vi "Actor Core.vi"(8 "error in":errorcluster, 11 "Image Acquisition in":refnum<class "Image Acquisition.lvclass">) -> (0 "error out":errorcluster, 3 "Actor out":refnum<class "Actor.lvclass">)   [LabVIEW 2019, in "Image Acquisition.lvlib" / "Image Acquisition.lvclass"]
doc: "(<B>Filename</B>: Actor Framework.lvlib:Actor.lvclass:Actor Core.vi)\n\nReceives messages to the actor, reacts to them, and initiates any error handling that may shut the actor down.\n\nDescendant classes may override this VI to append parallel tasks for the actor to complete while it handles messages. Overrides use the Call Parent Method node."
uses:
  Image Acquisition.lvclass
  <vilib>/ActorFramework/Actor/Actor.lvclass
  <vilib>/ActorFramework/Message Enqueuer/Message Enqueuer.lvclass
  Camera Controller/Camera Controller Messages/Child Handshake CC Msg/Child Handshake CC Msg.lvclass
  <vilib>/userdefined/High Color/IMAQdx.ctl
  <vilib>/vision/driver/IMAQdx.llb/IMAQdx Acquisition Mode.ctl
  <vilib>/vision/driver/IMAQdx.llb/IMAQdx Buffer Number Mode.ctl
  TypeDefs/Image Acquisition Parameters.ctl
  <vilib>/vision/Image Controls.llb/IMAQ Image.ctl
  TypeDefs/Initialize Data IA.ctl
  <resource>/objmgr/imaqdx.rc
  Camera Controller/Camera Controller Messages/Camera Information CC Msg/Camera Information CC Msg.lvclass
  <vilib>/event_ctls.llb/usereventprio.ctl
  Camera Controller/Camera Controller Messages/Get Image CC Msg/Get Image CC Msg.lvclass
  Camera Controller/Camera Controller Messages/State Acknowledgment CC Msg/State Acknowledgment CC Msg.lvclass
  C:/Program Files/National Instruments/LabVIEW 2019/vi.lib/ActorFramework/Actor/Actor.lvclass
panel:
  out "Image Acquisition ID":i32
  out "Acquired Image":T1(plugin-control)
  out "Camera Name":string
  out "Acquired Image Count":u64
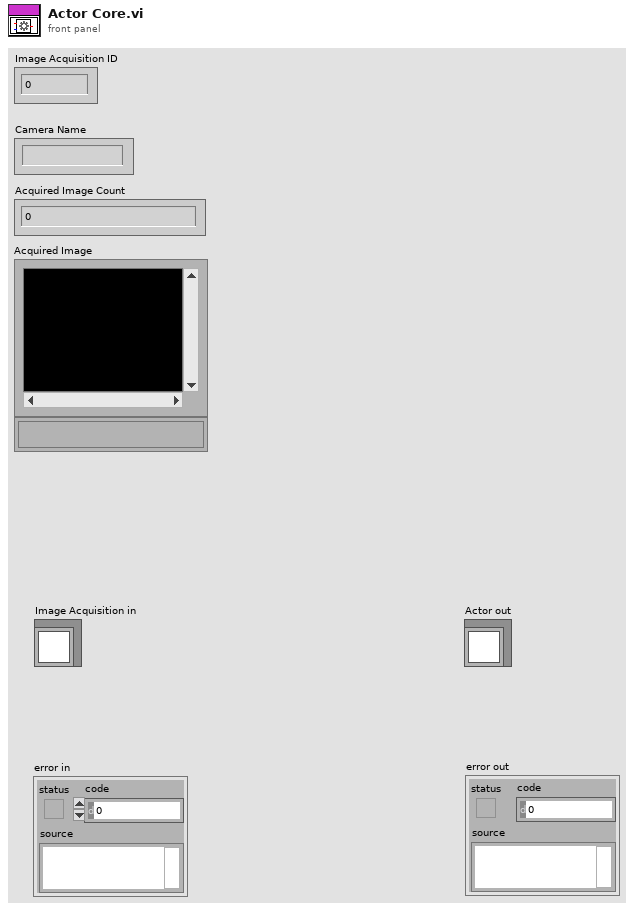
[diagram p1: front panel]
types:
  T1 = typedef "IMAQ Image.ctl" = refnum<image>
  T2 = typedef "Image Acquisition.lvlib/Image Acquisition.lvclass/Initialize Data IA.ctl" = cluster{"Core":cluster{"Current VI Reference":refnum<vi>, "Close Panel on Exit?":bool}, "IA JSON File Path":path, "Buffer Number":u64, "Missed Frame Count":i32, "Timeout":i32, "Image_Counter_CA":u64, "Imaqdx Session In":T3, "filenames":string[], "File path to read images":path, "Sequence":string, "IMAQ ring Buffer":T1[], "Buffer count":i32, "AOI":i32[], "Offline Images Ring Buffer":T1[], "ReceiverSequence":cluster{"ReceiverID":i32, "Index":i32}[], "Number Of Buffers":i32, "IMAQ Offline Image Buffer":T1[], "IMAQ Run image Buffer ":T1[], "Camera parameters":T4, "CurrentPartParameters":cluster{"Name":string, "ReceiverSequence":cluster{"ReceiverID":dbl, "Index":dbl}[], "AOI":i32[], "filePath":string}, "Exposure Time":u32, "File path @ Run":path, "State Ack":cluster{"State":string, "Status":string}}
  T3 = typedef "IMAQdx.ctl" = refnum<k21>
  T4 = typedef "Image Acquisition.lvlib/Image Acquisition.lvclass/Image Acquisition Parameters.ctl" = cluster{"Camera parameters":cluster{"Id":i32, "Type":string, "Model":string, "InterfaceType":string, "SerialNumber":string, "Timeout":i32, "NumberOfBuffers":i32, "AcquisitionTimeout":i32, "ImageName":string, "ColorCameraParam":cluster{"PixelFormat":string, "GammaEnable":bool, "GammaSelector":string, "BalanceRationSelector":string[], "BalanceRationRaw":i32[], "BalanceWhiteAuto":string, "LightSourceSelector":string}, "sessionID":T3, "Continuous?":T5, "Image Type":T6, "Buffer Number Mode (Next)":T7, "PartsList":cluster{"Name":string, "ReceiverSequence":cluster{"ReceiverID":dbl, "Index":dbl}[], "AOI":i32[], "filePath":string}[], "AOI ":i32[], "Default file path":path, "Offline":bool, "GeneralCameraConfig":cluster{"ActiveAttribute":string, "Value":string}[], "DefaultReceiverSequence":cluster{"ReceiverID":dbl, "Index":dbl}[], "Front Panel Open?":bool}, "PartName":string[]}
  T5 = typedef "NI_Vision_Acquisition_Software.lvlib/IMAQdx Acquisition Mode.ctl" = enum32{"One Shot", "Continuous"}
  T6 = typedef "Image Type" = u32
  T7 = typedef "NI_Vision_Acquisition_Software.lvlib/IMAQdx Buffer Number Mode.ctl" = enum32{"Next", "Last", "Buffer Number", "Every", "Last New"}
  T8 = typedef "Image Acquisition.lvlib/Image Acquisition.lvclass/Acquired Image Info.ctl" = cluster{"type":string, "Image Out":T1, "Buffer Number":u64, "Count":u64, "Buffer Count":u64}
  T9 = cluster{"Image out":T1, "Camera Location":string, "Count":u64, "RecieverSequence":cluster{"RecieverID":dbl, "Index":dbl}[]}
  T10 = enum32{"invalid app kind", "Development System", "Run Time System", "Student Edition", "Embedded LabVIEW", "Evaluation", "Custom"}
  T11 = enum32{"Invalid", "Standard", "Closed", "Hidden", "Minimized", "Maximized"}
  T12 = cluster{"Nested enqueuer":refnum<class "Message Enqueuer.lvclass">, "Clone name":string}
  T13 = cluster{"Camera Id":i32, "Camera Name":string, "Exposure Time":i32, "AOI":i32[]}
  T14 = typedef "usereventprio.ctl" = enum32{"high priority", "normal priority"}
  T15 = cluster{"ActiveAttribute":string, "Value":string}[]
  T16 = cluster{"ActiveAttribute":string, "Value":string}
  T17 = cluster{"Name":string, "ReceiverSequence":cluster{"ReceiverID":dbl, "Index":dbl}[], "AOI":i32[], "filePath":string}[]
  T18 = cluster{"Name":string, "ReceiverSequence":cluster{"ReceiverID":dbl, "Index":dbl}[], "AOI":i32[], "filePath":string}
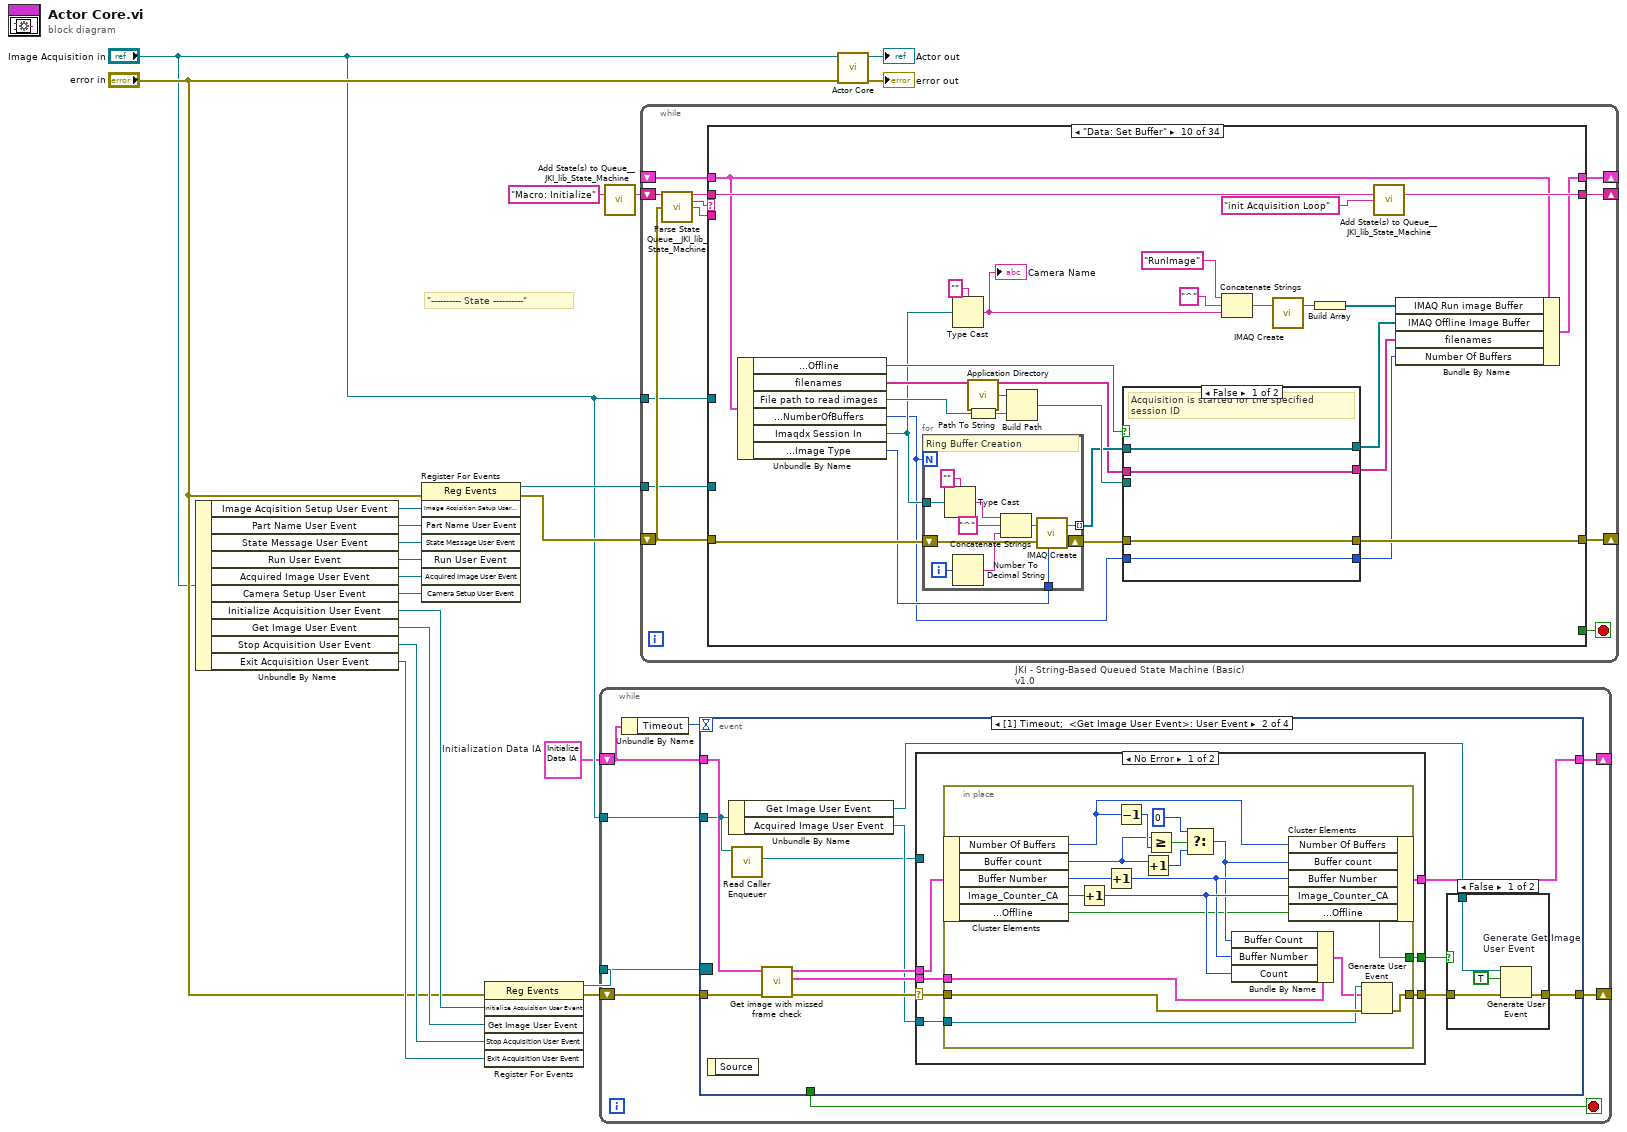
[diagram p0: block diagram]
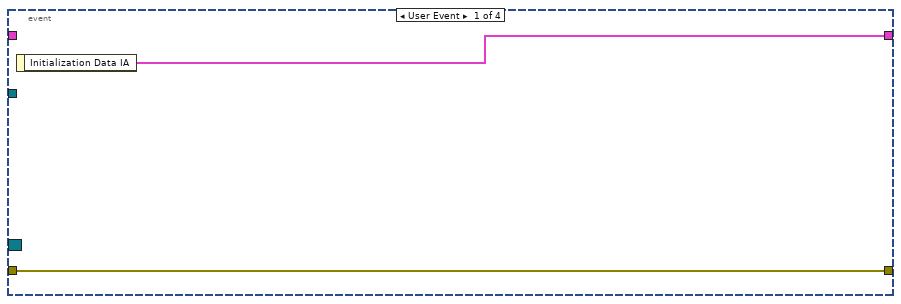
[diagram p2: hidden frame]
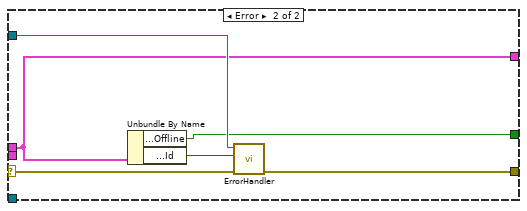
[diagram p4: hidden frame]
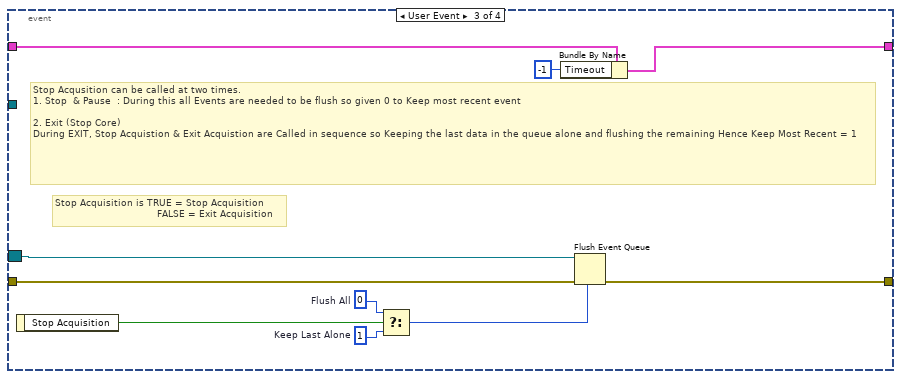
[diagram p5: hidden frame]
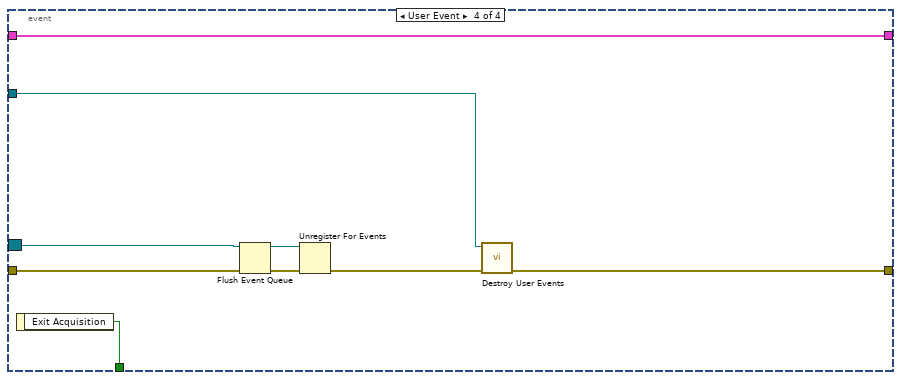
[diagram p6: hidden frame]
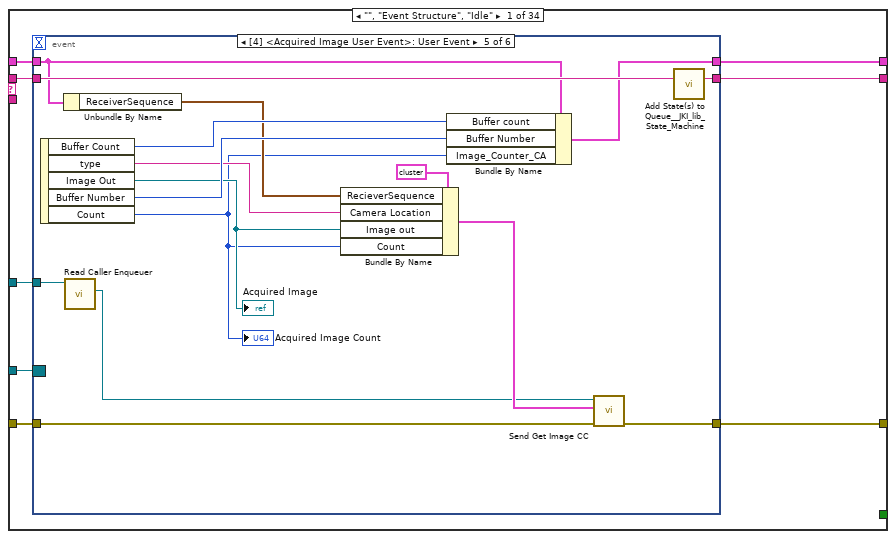
[diagram p7: hidden frame]
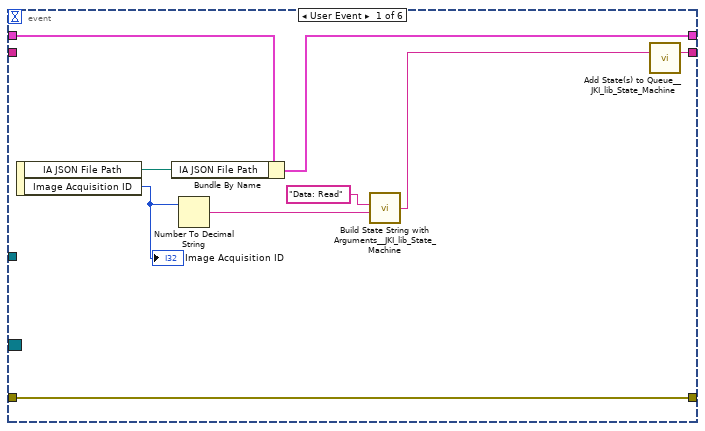
[diagram p8: hidden frame]
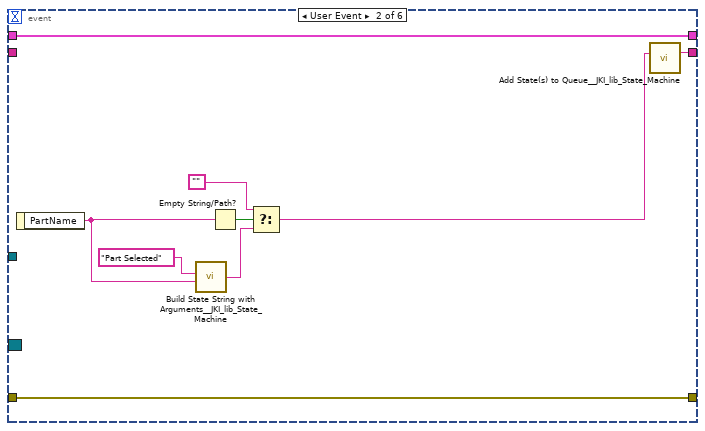
[diagram p9: hidden frame]
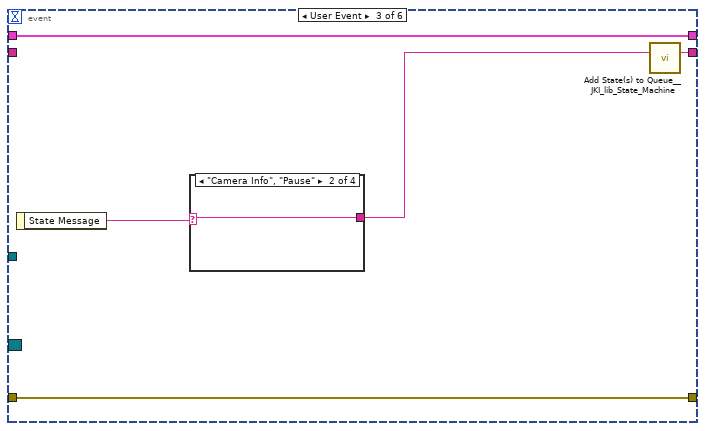
[diagram p10: hidden frame]
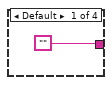
[diagram p11: hidden frame]
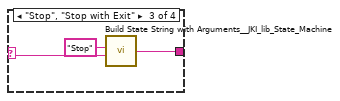
[diagram p12: hidden frame]
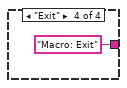
[diagram p13: hidden frame]
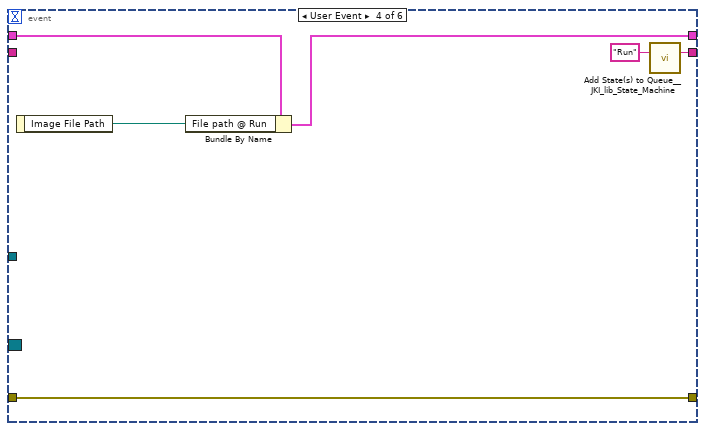
[diagram p14: hidden frame]
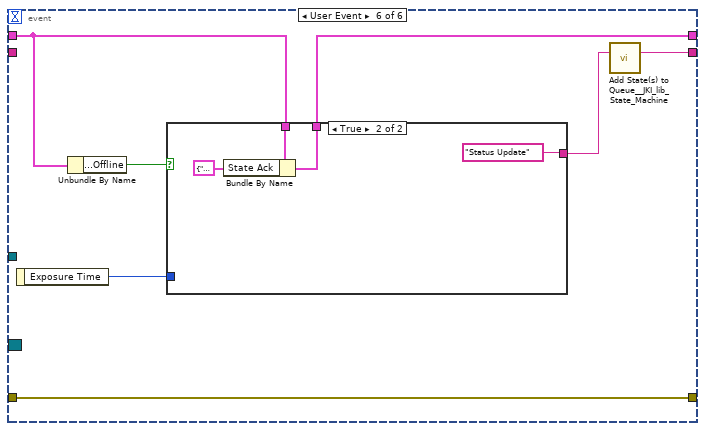
[diagram p15: hidden frame]
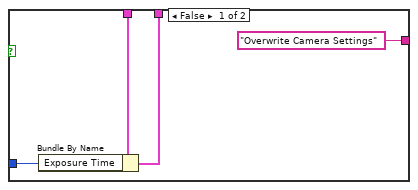
[diagram p16: hidden frame]
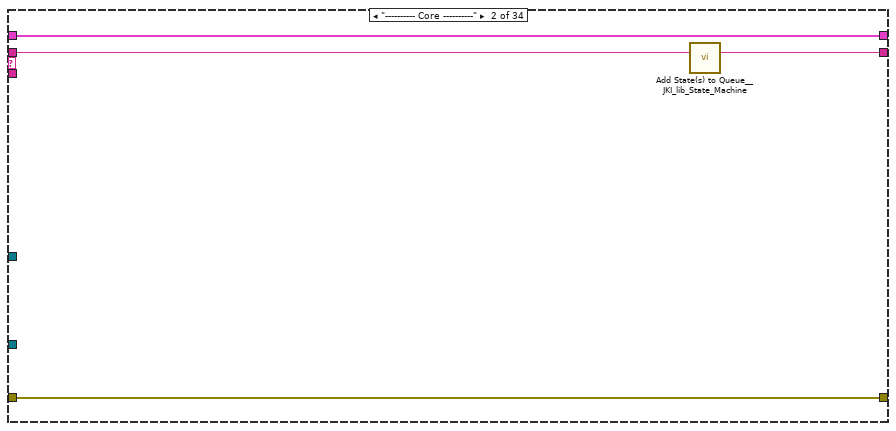
[diagram p17: hidden frame]
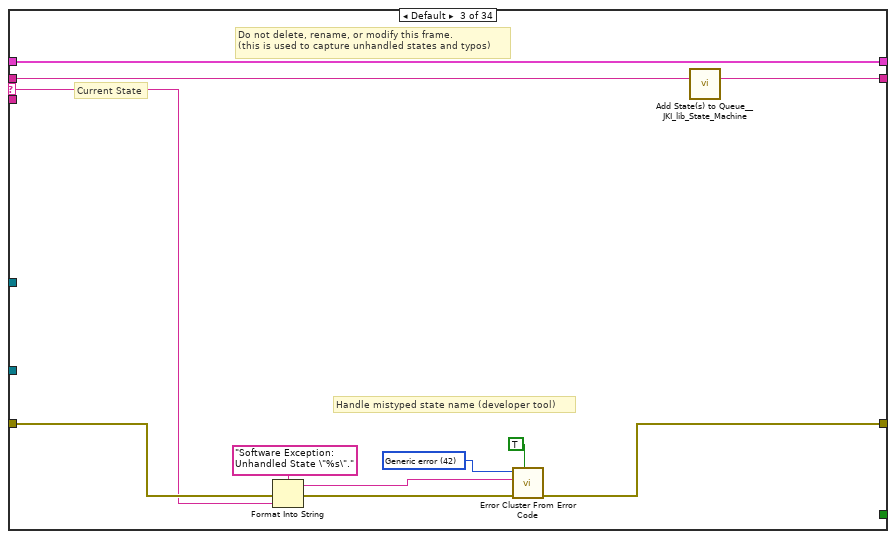
[diagram p18: hidden frame]
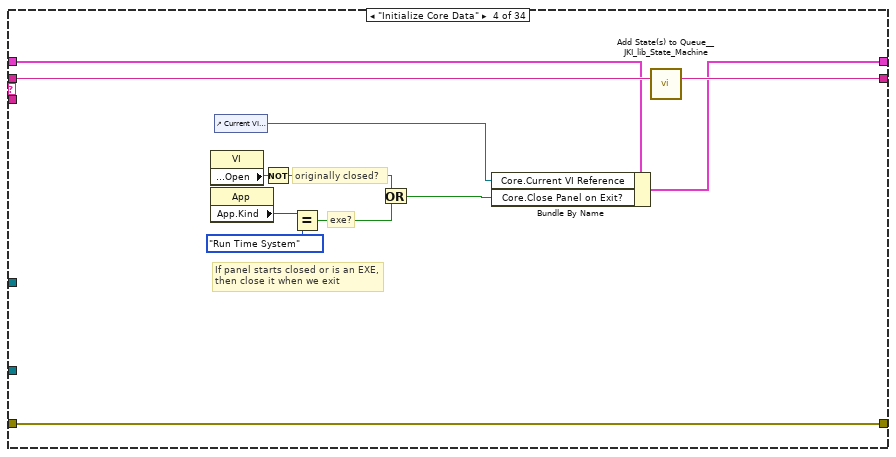
[diagram p19: hidden frame]
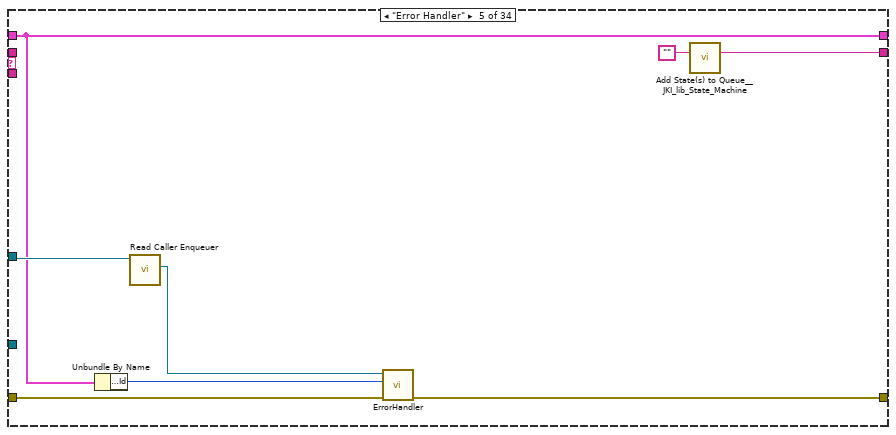
[diagram p20: hidden frame]
diagram:
  w1 = T2 {"Core"={"Current VI Reference"=refnum, "Close Panel on Exit?"=FALSE}, "IA JSON File Path"=path "", "Buffer Number"=0, "Missed Frame Count"=0, "Timeout"=-1, "Image_Counter_CA"=0, "Imaqdx Session In"="", "filenames"=[], "File path to read images"=path "", "Sequence"="", "IMAQ ring Buffer"=[], "Buffer count"=0, "AOI"=[], "Offline Images Ring Buffer"=[], "ReceiverSequence"=[], "Number Of Buffers"=0, "IMAQ Offline Image Buffer"=[], "IMAQ Run image Buffer "=[], "Camera parameters"={"Camera parameters"={"Id"=0, "Type"="", "Model"="", "InterfaceType"="", "SerialNumber"="", "Timeout"=0, "NumberOfBuffers"=0, "AcquisitionTimeout"=0, "ImageName"="", "ColorCameraParam"={"PixelFormat"="", "GammaEnable"=FALSE, "GammaSelector"="", "BalanceRationSelector"=[], "BalanceRationRaw"=[], "BalanceWhiteAuto"="", "LightSourceSelector"=""}, "sessionID"="", "Continuous?"=enum."One Shot", "Image Type"=0, "Buffer Number Mode (Next)"=enum."Next", "PartsList"=[{"Name"="", "ReceiverSequence"=[], "AOI"=[], "filePath"=""}], "AOI "=[], "Default file path"=path "", "Offline"=FALSE, "GeneralCameraConfig"=[], "DefaultReceiverSequence"=[], "Front Panel Open?"=FALSE}, "PartName"=[]}, "CurrentPartParameters"={"Name"="", "ReceiverSequence"=[], "AOI"=[], "filePath"=""}, "Exposure Time"=0, "File path @ Run"=path "", "State Ack"={"State"="", "Status"=""}}  # Initialization Data IA
  # "\"---------- State ----------\""
  n1 = Unbundle By Name("Image Acquisition in") -> ("Image Acqisition Setup User Event"=w17:refnum<user-event>, "Part Name User Event"=w16:refnum<user-event>, "State Message User Event"=w15:refnum<user-event>, "Run User Event"=w14:refnum<user-event>, "Acquired Image User Event"=w13:refnum<user-event>, "Camera Setup User Event"=w12:refnum<user-event>, "Initialize Acquisition User Event"=w9:refnum<user-event>, "Get Image User Event"=w8:refnum<user-event>, "Stop Acquisition User Event"=w7:refnum<user-event>, "Exit Acquisition User Event"=w6:refnum<user-event>)
  n2 = register-events(error in="error in", w17, w16, w15, w14, w13, w12) -> (reference out=w11:refnum<event-registration>, error out=w10:errorcluster)  [unwired: 1 in]
  n3 = register-events(error in="error in", w9, w8, w7, w6) -> (reference out=w5:refnum<event-registration>, error out=w3:errorcluster)  [unwired: 1 in]
  n4 = while {
    tunnel: w5 -> [w29]
    shift-right: [w26] -> _
    shift-left: w3 -> [w28]
    shift-right: [w27] -> _
    shift-left: w1 -> [w23]
    tunnel: "Image Acquisition in" -> [w24]
    stop <- w25 stop-if-true
    n5 = Unbundle By Name(w23) -> ("Timeout"=w22:i32)
    n6 = event shown="[1] Timeout;  <Get Image User Event>: User Event" {
      selector: w29 -> [_ _ w83 w93]
      dyn-events: _ -> [_ _ _ _]
      timeout: w22 -> [_ _ _ _]
      tunnel: w28 -> [w30 w44 w85 w94]
      tunnel: [w31 w32 w80 w98] -> w27
      tunnel: w23 -> [_ w43 w81 w98]
      tunnel: [w30 w37 w84 w91] -> w26
      tunnel: [_ _ _ w97] -> w25
      tunnel: w24 -> [_ w35 _ w90]
      event User Event {
        n7 = event-data() -> ("Initialization Data IA"=w31:T2)  [unwired: 1 in]
      }
      event Timeout; User Event {
        n8 = event-data() -> ()  [unwired: 1 in, 1 out]
        n9 = Unbundle By Name(w35) -> ("Get Image User Event"=w36:refnum<user-event>, "Acquired Image User Event"=w39:refnum<user-event>)
        n10 = call <vilib>:"Read Caller Enqueuer.vi"("Actor"=w35) -> ("Caller Enqueuer"=w34:refnum<class "Message Enqueuer.lvclass">)  [unwired: 10 in]
        n11 = call "Get image with missed frame check.vi"("error in"=w44, "Control IN"=w43) -> ("error out"=w42:errorcluster, "Get image Cluster"=w40:T8, "Controls Out"=w41:T2)  [unwired: 7 in]
        n12 = case shown="No Error" w42 {
          selector: w42 -> [w53 w79]
          tunnel: w41 -> [w56 w76]
          tunnel: w40 -> [w54 _]
          tunnel: [w55 w76] -> w32
          tunnel: w39 -> [w52 _]
          tunnel: [w51 w78] -> w38
          tunnel: w34 -> [_ w77]
          tunnel: [w50 w74] -> w33
          frame No Error {
            n13 = in-place {
              in-place-border: w54 -> [w58]
              in-place-border: w53 -> [w65]
              in-place-border: w52 -> [w63]
              in-place-border: [w64] -> w51
              in-place-border: [w57] -> w50
              n14 = in-place-cluster #1(w56) -> ("Number Of Buffers"=w66:i32, "Buffer count"=w69:i32, "Buffer Number"=w68:u64, "Image_Counter_CA"=w67:u64, "Camera parameters.Camera parameters.Offline"=w57:bool)
              n15 = Increment(x=w67) -> (x+1=w61:u64)
              n16 = Increment(x=w68) -> (x+1=w60:u64)
              n17 = Decrement(x=w66) -> (x-1=w72:i32)
              n18 = Increment(x=w69) -> (x+1=w70:i32)
              n19 = Greater Or Equal?(x=w69, y=w72) -> (x >= y?=w73:bool)
              n20 = Select(t=0, s=w73, f=w70) -> (s? t:f=w59:i32)
              n21 = Bundle By Name(cluster=w58, "Buffer Count"=w59, "Buffer Number"=w60, "Count"=w61) -> (w62:T8)
              n22 = in-place-cluster #1("Number Of Buffers"=w66, "Buffer count"=w59, "Buffer Number"=w60, "Image_Counter_CA"=w61, "Camera parameters.Camera parameters.Offline"=w57) -> (w55:T2)
              n23 = Generate User Event(user event=w63, event data cluster=w62, error in=w65) -> (error out=w64:errorcluster)  [unwired: 1 in, 1 out]
            }
          }
          frame Error {
            n24 = Unbundle By Name(w76) -> ("Camera parameters.Camera parameters.Offline"=w74:bool, "Camera parameters.Camera parameters.Id"=w75:i32)
            n25 = call "ErrorHandler.vi"("error in"=w79, "CameraID"=w75, "Caller Enqueuer"=w77) -> ("error out"=w78:errorcluster)  [unwired: 7 in, 1 out]
          }
        }
        n26 = case shown="False" w33 {
          tunnel: w38 -> [w48 w49]
          tunnel: [w47 w49] -> w37
          tunnel: w36 -> [w46 _]
          frame False {
            n27 = Generate User Event "Generate Get Image User Event"(user event=w46, event data cluster=TRUE ("event data"), error in=w48) -> (error out=w47:errorcluster)  [unwired: 1 in, 1 out]
          }
          frame True {
          }
        }
      }
      event User Event {
        w89 = 0  # Flush All
        w88 = 1  # Keep Last Alone
        # "Stop Acquisition is TRUE = Stop Acquisition\n                                  FALSE = Exit Acquisition"
        # "Stop Acqusition can be called at two times. \n1. Stop  & Pause  : During this all Events are needed to be flush so given 0 to Keep most recent event\n\n2. Exit (Stop Core)\nDuring EXIT, Stop Acquistion & Exit Acquistion are Called in sequence so Keeping the last data in the queue alone and flushing the remaining Hence Keep Most Recent = 1"
        n28 = event-data() -> ("Stop Acquisition"=w86:bool)  [unwired: 1 in]
        n29 = Select(t=w89, s=w86, f=w88) -> (s? t:f=w87:i32)
        n30 = Bundle By Name(cluster=w81, "Timeout"=-1) -> (w80:T2)
        n31 = Flush Event Queue(0:w83, 3:w85, 5:w87) -> (11:w84:errorcluster)  [unwired: 3 in, 2 out]
      }
      event User Event {
        n32 = event-data() -> ("Exit Acquisition"=w97:bool)  [unwired: 1 in]
        n33 = Flush Event Queue(0:w93, 3:w94) -> (8:w95:refnum<event-registration>, 11:w96:errorcluster)  [unwired: 4 in, 1 out]
        n34 = Unregister For Events(event registration refnum=w95, error in=w96) -> (error out=w92:errorcluster)
        n35 = call "Destroy User Events.vi"("error in (no error)"=w92, "Image Acquisition in"=w90) -> ("error out"=w91:errorcluster)  [unwired: 8 in, 1 out]
      }
    }
  }
  n36 = call <vilib>:"Add State(s) to Queue__JKI_lib_State_Machine.vi"("State(s) in (\"\")"="Macro: Initialize") -> ("States Out"=w19:string)  [unwired: 14 in]
  n37 = while "JKI - String-Based Queued State Machine (Basic) v1.0" {
    shift-right: [w103] -> _
    shift-left: _ -> [w102]
    shift-right: [w106] -> _
    shift-left: w10 -> [w101]
    shift-right: [w105] -> _
    shift-left: w19 -> [w107]
    tunnel: w11 -> [w100]
    tunnel: "Image Acquisition in" -> [w99]
    stop <- w104 stop-if-true
    n38 = call <vilib>:"Parse State Queue__JKI_lib_State_Machine.vi"("State Queue"=w107, "Error In (no error)"=w101) -> ("Remaining States"=w109:string, "Current State"=w110:string, "Arguments"=w108:string)  [unwired: 11 in]
    n39 = case shown="\"Data: Set Buffer\"" w110 {
      selector: w110 -> [_ _ w189 _ _ _ _ _ _ _ _ _ _ _ _ _ _ _ _ _ _ _ _ _ _ _ _ _ _ _ _ _ _ _]
      tunnel: w109 -> [w118 w188 w193 w211 _ w224 w228 w232 _ w288 w334 w350 w354 w360 w371 w397 w402 w414 w418 w430 w434 w449 _ _ _ w583 w627 w646 w680 w692 w700 w709 w717 w726]
      tunnel: w108 -> [_ _ _ _ _ _ _ _ w237 _ _ _ _ w355 w365 _ _ _ _ _ _ _ w459 _ _ w560 _ _ _ _ _ _ _ _]
      tunnel: w102 -> [w116 w185 w191 w202 w215 w222 w225 _ w235 w275 w330 w347 w352 w358 w367 w394 w399 w412 w415 w428 w431 w442 w454 w495 w544 w567 w624 w630 w663 w689 w694 w702 w715 w724]
      tunnel: [w115 w186 w195 w208 w213 w221 w226 w230 w239 w284 w324 w348 w351 w356 w368 w395 w400 w404 w416 w422 w432 w446 w456 w505 w545 w581 w625 w634 errorcluster {"status"=FALSE, "code"=0, "source"=""} ("error in (no error)") w690 w697 w705 w713 w722] -> w106
      tunnel: w101 -> [w114 w186 w194 w208 w218 w221 w226 w230 w240 w285 w331 w348 w351 w357 w369 w395 w400 w405 w416 w424 w432 w447 w457 w506 w546 w563 w625 w644 w672 w690 _ w706 w714 w723]
      tunnel: [w117 w187 w192 w210 w219 w223 w227 w231 w233 w287 w333 w349 w353 w359 w370 w396 w401 w413 w417 w429 w433 w448 w460 w507 w554 w582 w626 w645 w679 w691 w699 w708 w716 w725] -> w105
      tunnel: [_ _ _ _ _ TRUE _ _ _ _ _ _ _ _ _ _ _ _ _ _ _ _ _ _ _ _ _ _ _ _ _ _ _ _] -> w104
      tunnel: [w113 w185 w191 w209 w215 w222 w225 w229 w234 w274 w330 w347 w352 w358 w367 w394 w399 w412 w415 w428 w431 w442 w458 w494 w544 w580 w624 w629 w664 w689 w694 w702 w715 w724] -> w103
      tunnel: w100 -> [w112 _ _ _ _ _ _ _ _ _ _ _ _ _ _ _ _ w403 _ _ _ _ _ _ _ _ _ _ _ _ _ _ _ _]
      tunnel: w99 -> [w111 _ _ _ w217 _ _ _ _ _ _ _ _ _ _ _ _ _ _ w421 _ w445 _ _ w547 w564 _ w640 _ _ w696 w707 w712 w721]
      frame "", "Event Structure", "Idle" {
        n40 = event shown="[4] <Acquired Image User Event>: User Event" {
          selector: w112 -> [_ _ _ _ _ _]
          dyn-events: _ -> [_ _ _ _ _ _]
          timeout: _ -> [_ _ _ _ _ _]
          tunnel: w118 -> [_ _ _ _ w169 _]
          tunnel: [w127 w136 w141 w153 w168 w176] -> w117
          tunnel: w116 -> [w124 w134 w139 w150 w162 w171]
          tunnel: [w126 w135 w140 w152 w157 w175] -> w115
          tunnel: w114 -> [w126 w135 w140 w152 w158 w175]
          tunnel: [w123 w134 w139 w149 w161 w173] -> w113
          tunnel: w111 -> [_ _ _ _ w156 _]
          event User Event {
            n41 = event-data() -> ("IA JSON File Path"=w125:path, "Image Acquisition ID"=w122:i32)  [unwired: 1 in]
            "Image Acquisition ID" <- w122
            n42 = Bundle By Name(cluster=w124, "IA JSON File Path"=w125) -> (w123:T2)
            n43 = Number To Decimal String(number=w122) -> (decimal integer string=w121:string)  [unwired: 1 in]
            n44 = call <vilib>:"Build State String with Arguments__JKI_lib_State_Machine.vi"("Arguments (\"\")"=w121, "State"="Data: Read") -> ("State with Arguments"=w119:string)  [unwired: 4 in]
            n45 = call <vilib>:"Add State(s) to Queue__JKI_lib_State_Machine.vi"("State(s) in (\"\")"=w119) -> ("States Out"=w127:string)  [unwired: 14 in]
          }
          event User Event {
            n46 = event-data() -> ("PartName"=w133:string)  [unwired: 1 in]
            n47 = call <vilib>:"Build State String with Arguments__JKI_lib_State_Machine.vi"("Arguments (\"\")"=w133, "State"="Part Selected") -> ("State with Arguments"=w130:string)  [unwired: 4 in]
            n48 = Empty String/Path?(string/path=w133) -> (empty?=w132:bool)
            n49 = Select(t="", s=w132, f=w130) -> (s? t:f=w128:string)
            n50 = call <vilib>:"Add State(s) to Queue__JKI_lib_State_Machine.vi"("State(s) in (\"\")"=w128) -> ("States Out"=w136:string)  [unwired: 14 in]
          }
          event User Event {
            n51 = event-data() -> ("State Message"=w138:string)  [unwired: 1 in]
            n52 = case shown="\"Camera Info\", \"Pause\"" w138 {
              selector: w138 -> [_ w143 w146 _]
              tunnel: ["" w143 w144 "Macro: Exit" ("State with Arguments")] -> w137
              frame Default {
              }
              frame "Camera Info", "Pause" {
              }
              frame "Stop", "Stop with Exit" {
                n53 = call <vilib>:"Build State String with Arguments__JKI_lib_State_Machine.vi"("Arguments (\"\")"=w146, "State"="Stop") -> ("State with Arguments"=w144:string)  [unwired: 4 in]
              }
              frame "Exit" {
              }
            }
            n54 = call <vilib>:"Add State(s) to Queue__JKI_lib_State_Machine.vi"("State(s) in (\"\")"=w137) -> ("States Out"=w141:string)  [unwired: 14 in]
          }
          event User Event {
            n55 = event-data() -> ("Image File Path"=w151:path)  [unwired: 1 in]
            n56 = Bundle By Name(cluster=w150, "File path @ Run"=w151) -> (w149:T2)
            n57 = call <vilib>:"Add State(s) to Queue__JKI_lib_State_Machine.vi"("State(s) in (\"\")"="Run" ("State(s) in (\"\")")) -> ("States Out"=w153:string)  [unwired: 14 in]
          }
          event User Event {
            n58 = event-data() -> ("Buffer Count"=w164:u64, "type"=w165:string, "Image Out"=w166:T1, "Buffer Number"=w167:u64, "Count"=w154:u64)  [unwired: 1 in]
            "Acquired Image Count" <- w154
            "Acquired Image" <- w166
            n59 = Unbundle By Name(w162) -> ("ReceiverSequence"=w163:cluster{"ReceiverID":i32, "Index":i32}[])
            n60 = call <vilib>:"Read Caller Enqueuer.vi"("Actor"=w156) -> ("Caller Enqueuer"=w155:refnum<class "Message Enqueuer.lvclass">)  [unwired: 10 in]
            n61 = Bundle By Name(cluster=T9 {"Image out"=refnum, "Camera Location"="", "Count"=0, "RecieverSequence"=[]} ("Acquired Image Info"), "RecieverSequence"=w163, "Camera Location"=w165, "Image out"=w166, "Count"=w154) -> (w159:T9)
            n62 = Bundle By Name(cluster=w162, "Buffer count"=w164, "Buffer Number"=w167, "Image_Counter_CA"=w154) -> (w161:T2)
            n63 = call "Send Get Image CC.vi"("error in (no error)"=w158, "Acquired Image Info"=w159, "Message Enqueuer"=w155) -> ("error out"=w157:errorcluster)  [unwired: 7 in, 1 out]
            n64 = call <vilib>:"Add State(s) to Queue__JKI_lib_State_Machine.vi"("State(s) in (\"\")"=w169) -> ("States Out"=w168:string)  [unwired: 14 in]
          }
          event User Event {
            n65 = event-data() -> ("Exposure Time"=w174:i32)  [unwired: 1 in]
            n66 = Unbundle By Name(w171) -> ("Camera parameters.Camera parameters.Offline"=w170:bool)
            n67 = case shown="True" w170 {
              tunnel: w174 -> [w180 _]
              tunnel: [w179 w182] -> w173
              tunnel: ["Overwrite Camera Settings" "Status Update"] -> w172
              tunnel: w171 -> [w177 w183]
              frame False {
                n68 = Bundle By Name(cluster=w177, "Exposure Time"=w180) -> (w179:T2)
              }
              frame True {
                n69 = Bundle By Name(cluster=w183, "State Ack"=cluster{"State":string, "Status":string} {"State"="Setup", "Status"="Fail"}) -> (w182:T2)
              }
            }
            n70 = call <vilib>:"Add State(s) to Queue__JKI_lib_State_Machine.vi"("State(s) in (\"\")"=w172) -> ("States Out"=w176:string)  [unwired: 14 in]
          }
        }
      }
      frame "---------- Core ----------" {
        n71 = call <vilib>:"Add State(s) to Queue__JKI_lib_State_Machine.vi"("State(s) in (\"\")"=w188) -> ("States Out"=w187:string)  [unwired: 14 in]
      }
      frame Default {
        w198 = 42 items=["No error", "Argument error", "Memory is full", "Out of zone", "End of file", "File already open", "Generic file I/O error", "File not found", "File permission error", "Disk is full", "Duplicate path", "Too many files open", "System feature not enabled", "Resource file not found", "Cannot add resource", "Resource not found", "Image not found", "Image memory error", "Pen does not exist", "Config type invalid", "Config token not found", "Config parse error", "Config memory error", "Bad external code format", "Bad external code offset", "External code not present", "Null window", "Destroy window error", "Null menu", "Print aborted", "Bad print record", "Print driver error", "Windows error during printing", "Memory error during printing", "Print dialog error", "Generic print error", "Invalid device refnum", "Device not found", "Device parameter error", "Device unit error", "Cannot open device", "Device call aborted", "Generic error", "Cancelled by user", "Object ID too low", "Object ID too high", "Object not in heap", "Unknown heap", "Unknown object (invalid DefProc)", "Unknown object (DefProc not in table)", "Message out of range", "Invalid (null) method", "Unknown message", "Manager call not supported", "Bad address", "Network operation in progress", "Network operation timed out", "Connection is busy", "Network attribute not supported", "Network error", "Address in use", "System out of memory", "Connection aborted", "Connection refused", "Not connected", "Already connected", "Connection closed", "Initialization error (interapplication manager)", "Bad occurrence", "Wait on unbound occurrence handler", "Occurrence queue overflow", "Datalog type conflict", "Unused", "Unrecognized type (interapplication manager)", "Memory corrupt", "Failed to make temporary DLL", "Old CIN version", "Drag socket not found", "Failed to load drop-object", "Failed to register OLE object", "Failed to release OLE object", "Format specifier type mismatch", "Unknown format specifier", "Too few format specifiers", "Too many format specifiers", "Scan failed", "Newer CIN version", "Error converting to variant", "Runtime menu error", "Password tampered", "Variant attribute not found", "Incompatible variant data type", "Event data is not available", "Event Store is not present", "Occurrence is not found", "Event Queue is not created", "Event info is not available", "Refnum passed is NULL", "Error retrieving Class GUID", "Error retrieving CoClass GUID", "Error retrieving TypeLib GUID.", "Bad built application magic bytes.", "Specific driver is different from the specific driver associated with the Logical Name.", "There is no session opened to the class driver.", "Max Error", "MAX - Error with config objects", "MAX - Error loading configuration", "MAX - Group not supported"]
        # "Current State"
        # "Do not delete, rename, or modify this frame.\n(this is used to capture unhandled states and typos)"
        # "Handle mistyped state name (developer tool)"
        n72 = Format Into String(format string="Software Exception: Unhandled State \"%s\"." ("message"), error in=w194, w189) -> (resulting string=w197:string, error out=w196:errorcluster)  [unwired: 1 in]
        n73 = call <vilib>:"Error Cluster From Error Code.vi"("show call chain? (False)"=TRUE, "error in (no error)"=w196, "error message (\"\")"=w197, "error code (0)"=w198) -> ("error out"=w195:errorcluster)  [unwired: 5 in]
        n74 = call <vilib>:"Add State(s) to Queue__JKI_lib_State_Machine.vi"("State(s) in (\"\")"=w193) -> ("States Out"=w192:string)  [unwired: 14 in]
      }
      frame "Initialize Core Data" {
        # "originally closed?"
        # "exe?"
        # "If panel starts closed or is an EXE, then close it when we exit"
        n75 = property class="VI"() -> ("Front Panel.Open"=w207:bool)  [unwired: 2 in, 2 out]
        n76 = property class="App"() -> ("App.Kind"=w206:T10)  [unwired: 2 in, 2 out]
        n77 = control-ref of="Current VI Reference"() -> (w200:refnum<vi>)
        n78 = Not(x=w207) -> (.not. x?=w204:bool)
        n79 = Equal?(x=w206, y=T10."Run Time System" ("Application:Kind")) -> (x = y?=w203:bool)
        n80 = Or(x=w204, y=w203) -> (x .or. y?=w201:bool)
        n81 = Bundle By Name(cluster=w202, "Core.Current VI Reference"=w200, "Core.Close Panel on Exit?"=w201) -> (w209:T2)
        n82 = call <vilib>:"Add State(s) to Queue__JKI_lib_State_Machine.vi"("State(s) in (\"\")"=w211) -> ("States Out"=w210:string)  [unwired: 14 in]
      }
      frame "Error Handler" {
        n83 = Unbundle By Name(w215) -> ("Camera parameters.Camera parameters.Id"=w214:i32)
        n84 = call <vilib>:"Read Caller Enqueuer.vi"("Actor"=w217) -> ("Caller Enqueuer"=w216:refnum<class "Message Enqueuer.lvclass">)  [unwired: 10 in]
        n85 = call "ErrorHandler.vi"("error in"=w218, "CameraID"=w214, "Caller Enqueuer"=w216) -> ("error out"=w213:errorcluster)  [unwired: 7 in, 1 out]
        n86 = call <vilib>:"Add State(s) to Queue__JKI_lib_State_Machine.vi"("State(s) in (\"\")"="") -> ("States Out"=w219:string)  [unwired: 14 in]
      }
      frame "Exit" {
        # "Do not put any code in this frame.\n(No errors that occur here will be handled.)"
        n87 = call <vilib>:"Add State(s) to Queue__JKI_lib_State_Machine.vi"("State(s) in (\"\")"=w224) -> ("States Out"=w223:string)  [unwired: 14 in]
      }
      frame "---------- Data ----------" {
        # "Do not put any code in this frame.\n(It is a separator no-op. You can make a copy of this frame to create a new Data frame)"
        n88 = call <vilib>:"Add State(s) to Queue__JKI_lib_State_Machine.vi"("State(s) in (\"\")"=w228) -> ("States Out"=w227:string)  [unwired: 14 in]
      }
      frame "Data: Initialize" {
        w229 = T2 {"Core"={"Current VI Reference"=refnum, "Close Panel on Exit?"=FALSE}, "IA JSON File Path"=path "", "Buffer Number"=0, "Missed Frame Count"=0, "Timeout"=-1, "Image_Counter_CA"=0, "Imaqdx Session In"="", "filenames"=[], "File path to read images"=path "", "Sequence"="", "IMAQ ring Buffer"=[], "Buffer count"=0, "AOI"=[], "Offline Images Ring Buffer"=[], "ReceiverSequence"=[], "Number Of Buffers"=0, "IMAQ Offline Image Buffer"=[], "IMAQ Run image Buffer "=[], "Camera parameters"={"Camera parameters"={"Id"=0, "Type"="", "Model"="", "InterfaceType"="", "SerialNumber"="", "Timeout"=0, "NumberOfBuffers"=0, "AcquisitionTimeout"=0, "ImageName"="", "ColorCameraParam"={"PixelFormat"="", "GammaEnable"=FALSE, "GammaSelector"="", "BalanceRationSelector"=[], "BalanceRationRaw"=[], "BalanceWhiteAuto"="", "LightSourceSelector"=""}, "sessionID"="", "Continuous?"=enum."One Shot", "Image Type"=0, "Buffer Number Mode (Next)"=enum."Next", "PartsList"=[{"Name"="", "ReceiverSequence"=[], "AOI"=[], "filePath"=""}], "AOI "=[], "Default file path"=path "", "Offline"=FALSE, "GeneralCameraConfig"=[], "DefaultReceiverSequence"=[], "Front Panel Open?"=FALSE}, "PartName"=[]}, "CurrentPartParameters"={"Name"="", "ReceiverSequence"=[], "AOI"=[], "filePath"=""}, "Exposure Time"=0, "File path @ Run"=path "", "State Ack"={"State"="", "Status"=""}}  # Initialization Data IA
        n89 = call <vilib>:"Add State(s) to Queue__JKI_lib_State_Machine.vi"("State(s) in (\"\")"=w232) -> ("States Out"=w231:string)  [unwired: 14 in]
      }
      frame "Data: Read" {
        n90 = Unbundle By Name(w235) -> ("IA JSON File Path"=w238:path)
        n91 = call "ReadJSONImageAcquisitionParameters.vi"("error in"=w240, "Camera ID"=w237, "file path (use dialog)"=w238) -> ("error out"=w239:errorcluster, "Camera parameters"=w236:T4)  [unwired: 7 in]
        n92 = in-place {
          in-place-border: w236 -> [w260]
          in-place-border: [w252] -> w233
          n93 = in-place-cluster #2(w235) -> ()  [unwired: 6 out]
          n94 = in-place-cluster #3(w236) -> ("Camera parameters.GeneralCameraConfig"=w242:T15, "Camera parameters.sessionID"=w246:T3, "Camera parameters.Front Panel Open?"=w251:bool, "Camera parameters.Offline"=w250:bool, "Camera parameters.Default file path"=w249:path, "Camera parameters.DefaultReceiverSequence"=w248:cluster{"ReceiverID":dbl, "Index":dbl}[], "Camera parameters.AOI"=w247:i32[])
          n95 = Index Array(array=w242, index=2) -> (element=w244:T16)
          n96 = Unbundle By Name(w244) -> ("Value"=w243:string)
          n97 = Select(t="UI: Front Panel State >> Open ", s=w251, f="UI: Front Panel State >> Close ") -> (s? t:f=w255:string)
          n98 = Decimal String To Number(string=w243) -> (number=w241:i32)  [unwired: 2 in, 1 out]
          n99 = Select(t="", s=w250, f="Set Camera Properties") -> (s? t:f=w254:string)
          n100 = in-place-cluster #3("Camera parameters.GeneralCameraConfig"=w242, "Camera parameters.sessionID"=w246, "Camera parameters.Front Panel Open?"=w251, "Camera parameters.Offline"=w250, "Camera parameters.Default file path"=w249, "Camera parameters.DefaultReceiverSequence"=w248, "Camera parameters.AOI"=w247) -> ()  [unwired: 1 out]
          n101 = in-place-cluster #2("File path to read images"=w249, "ReceiverSequence"=w248, "AOI"=w247, "Camera parameters"=w260, "Imaqdx Session In"=w246, "Exposure Time"=w241) -> (w234:T2)
          n102 = call <vilib>:"Add State(s) to Queue__JKI_lib_State_Machine.vi"("State(s) in Front (\"\")"=w255, "State(s) in (\"\")"=w254, "State(s) at Back (\"\")"="Data: Set Buffer" ("State(s) in (\"\")")) -> ("States Out"=w252:string)  [unwired: 12 in]
        }
      }
      frame "Data: Set Buffer" {
        n103 = Unbundle By Name(w275) -> ("Camera parameters.Camera parameters.Offline"=w278:bool, "filenames"=w277:string[], "File path to read images"=w281:path, "Camera parameters.Camera parameters.NumberOfBuffers"=w262:i32, "Imaqdx Session In"=w267:T3, "Camera parameters.Camera parameters.Image Type"=w276:T6)
        n104 = for {
          N: w262 -> [_]
          shift-right: [w320] -> w286
          shift-left: w285 -> [w321]
          tunnel: w267 -> [w317]
          tunnel: w276 -> [w312]
          tunnel: [w311] -> w279 mode=indexing
          i -> [w314]
          # "Ring Buffer Creation"
          n105 = Type Cast(type="" ("Camera Location"), x=w317) -> (*(type *) &x=w319:string)
          n106 = Number To Decimal String(number=w314) -> (decimal integer string=w313:string)  [unwired: 1 in]
          n107 = Concatenate Strings(w319, "^" ("string"), w313) -> (w315:string)
          n108 = call "IMAQ Create"("Image Name"=w315, "Image Type"=w312, "error in (no error)"=w321) -> ("New Image"=w311:T1, "error out"=w320:errorcluster)  [unwired: 2 in]
        }
        n109 = Type Cast(type="" ("Camera Location"), x=w267) -> (*(type *) &x=w265:string)
        "Camera Name" <- w265
        n110 = call <vilib>:"Application Directory.vi"() -> ("Application Directory"=w283:path)
        n111 = Path To String(path=w281) -> (string=w282:string)
        n112 = Build Path(base path=w283, name or relative path=w282) -> (appended path=w280:path)
        n113 = case shown="False" w278 {
          tunnel: w286 -> [w292 w302]
          tunnel: [w292 w297] -> w284
          tunnel: w280 -> [_ w300]
          tunnel: w277 -> [w290 _]
          tunnel: w279 -> [w291 w294]
          tunnel: [w291 w296] -> w269
          tunnel: [w290 w295] -> w271
          tunnel: [w289 w293] -> w261
          tunnel: w262 -> [w289 _]
          frame False {
            # "Acquisition is started for the specified session ID"
          }
          frame True {
            # "database is accessed for the image names and sorted"
            n114 = List Folder(path=w300, error in=w302) -> (filenames=w301:string[], error out=w298:errorcluster)  [unwired: 2 in, 2 out]
            n115 = Sort 1D Array ("Sort Array")(array=w301) -> (sorted array=w299:string[])
            n116 = for {
              tunnel: w300 -> [w310]
              tunnel: w299 -> [w306] mode=indexing
              shift-right: [w309] -> w297
              shift-left: w298 -> [w305]
              tunnel: [w307] -> w296 mode=indexing
              tunnel: [w306] -> w295 mode=indexing
              tunnel: w294 -> [w304] mode=indexing
              tunnel: [w303] -> w293
              i -> [w303]
              n117 = Build Path(base path=w310, name or relative path=w306) -> (appended path=w308:path)
              n118 = call "IMAQ ReadFile"("File Path"=w308, "error in (no error)"=w305, "Image"=w304) -> ("error out"=w309:errorcluster, "Image Out"=w307:T1)  [unwired: 4 in, 3 out]
            }
          }
        }
        n119 = Concatenate Strings("RunImage" ("Image Name"), "^" ("string"), w265) -> (w263:string)
        n120 = call "IMAQ Create"("Image Name"=w263) -> ("New Image"=w273:T1)  [unwired: 4 in, 1 out]
        n121 = Build Array(w273) -> (w272:T1[])
        n122 = call <vilib>:"Add State(s) to Queue__JKI_lib_State_Machine.vi"("State(s) in (\"\")"=w288, "State(s) at Back (\"\")"="init Acquisition Loop" ("State(s) at Back (\"\")")) -> ("States Out"=w287:string)  [unwired: 13 in]
        n123 = Bundle By Name(cluster=w275, "IMAQ Run image Buffer"=w272, "IMAQ Offline Image Buffer"=w269, "filenames"=w271, "Number Of Buffers"=w261) -> (w274:T2)
      }
      frame "Data: Cleanup" {
        n124 = Unbundle By Name(w330) -> ("IMAQ Offline Image Buffer"=w323:T1[], "IMAQ Run image Buffer"=w322:T1[], "Imaqdx Session In"=w328:T3, "Camera parameters.Camera parameters.Offline"=w327:bool, "Core.Current VI Reference"=w332:refnum<vi>)
        n125 = Close Reference(reference=w332, error in (no error)=w331) -> (error out=w329:errorcluster)
        n126 = case shown="False" w327 {
          tunnel: w329 -> [w341 w346]
          tunnel: w328 -> [w342 _]
          tunnel: [w344 w346] -> w325
          frame False {
            n127 = call <vilib>:"IMAQdx Unconfigure Acquisition.vi"("error in"=w341, "Session In"=w342) -> ("error out"=w345:errorcluster, "Session Out"=w343:T3)  [unwired: 8 in]
            n128 = call <vilib>:"IMAQdx Close Camera.vi"("error in"=w345, "Session In"=w343) -> ("error out"=w344:errorcluster)  [unwired: 9 in]
          }
          frame True {
          }
        }
        n129 = call <vilib>:"Add State(s) to Queue__JKI_lib_State_Machine.vi"("State(s) in (\"\")"=w334) -> ("States Out"=w333:string)  [unwired: 14 in]
        n130 = for {
          tunnel: [w340] -> w326
          tunnel: w322 -> [w339] mode=indexing
          tunnel: w325 -> [w338]
          n131 = call "IMAQ Dispose"("Image"=w339, "error in (no error)"=w338) -> ("error out"=w340:errorcluster)  [unwired: 4 in]
        }
        n132 = for {
          tunnel: w326 -> [w337]
          tunnel: w323 -> [w335] mode=indexing
          tunnel: [w336] -> w324
          tunnel: [w335] -> _ mode=indexing
          n133 = call "IMAQ Dispose"("Image"=w335, "error in (no error)"=w337) -> ("error out"=w336:errorcluster)  [unwired: 4 in]
        }
      }
      frame "---------- UI ----------" {
        n134 = call <vilib>:"Add State(s) to Queue__JKI_lib_State_Machine.vi"("State(s) in (\"\")"=w350) -> ("States Out"=w349:string)  [unwired: 14 in]
      }
      frame "UI: Initialize" {
        # "Initialize the User Interface, here.\n(this is called automatically, by the Macro: Init)"
        n135 = call <vilib>:"Add State(s) to Queue__JKI_lib_State_Machine.vi"("State(s) in (\"\")"=w354) -> ("States Out"=w353:string)  [unwired: 14 in]
      }
      frame "UI: Cursor Set" {
        # "Argument"
        # "Set and Unset Cursor Busy.\n(Usage: \"UI: Cursor Set >> Busy|Idle\")"
        n136 = case shown="\"Idle\", Default" w355 {
          tunnel: w357 -> [w362 w364]
          tunnel: [w361 w363] -> w356
          frame "Idle", Default {
            n137 = call <vilib>:"Unset Busy.vi"("error in (no error)"=w362) -> ("error out"=w361:errorcluster)  [unwired: 10 in]
          }
          frame "Busy" {
            n138 = call <vilib>:"Set Busy.vi"("error in (no error)"=w364) -> ("error out"=w363:errorcluster)  [unwired: 9 in, 1 out]
          }
        }
        n139 = call <vilib>:"Add State(s) to Queue__JKI_lib_State_Machine.vi"("State(s) in (\"\")"=w360) -> ("States Out"=w359:string)  [unwired: 14 in]
      }
      frame "UI: Front Panel State" {
        # "Argument"
        # "Set Front Panel Open or Closed\n(Usage: \"UI: Front Panel State >> Open|Close\")"
        n140 = Unbundle By Name(w367) -> ("Core.Current VI Reference"=w366:refnum<vi>)
        n141 = case shown="\"Open\", Default" w365 {
          tunnel: w369 -> [w375 w388]
          tunnel: [w377 w389] -> w368
          tunnel: w366 -> [w376 w386]
          frame "Open", Default {
            n142 = property class="VI"(reference=w376, error in=w375) -> (reference out=w373:refnum<vi>, error out=w374:errorcluster, "Front Panel.Open"=w372:bool)
            n143 = case shown="False" w372 {
              tunnel: [w380 w383] -> w377
              tunnel: w374 -> [w379 w383]
              tunnel: w373 -> [w378 _]
              frame False {
                n144 = invoke class="VI" method="FP.Open"(reference=w378, error in=w379, "Activate"=TRUE, "State"=T11."Standard") -> (error out=w380:errorcluster)  [unwired: 1 in, 4 out]
              }
              frame True {
              }
            }
          }
          frame "Close" {
            n145 = property class="VI"(reference=w386, error in=w388) -> (reference out=w385:refnum<vi>, error out=w387:errorcluster, "Front Panel.Open"=w384:bool)
            n146 = case shown="True" w384 {
              tunnel: [w390 w393] -> w389
              tunnel: w387 -> [w390 w392]
              tunnel: w385 -> [_ w391]
              frame False {
              }
              frame True {
                n147 = invoke class="VI" method="FP.Close"(reference=w391, error in=w392) -> (error out=w393:errorcluster)  [unwired: 1 in, 2 out]
              }
            }
          }
        }
        n148 = call <vilib>:"Add State(s) to Queue__JKI_lib_State_Machine.vi"("State(s) in (\"\")"=w371) -> ("States Out"=w370:string)  [unwired: 14 in]
      }
      frame "---------- Macro ----------" {
        # "Do not put any code in this frame.\n(It is a separator no-op. You can make a copy of this frame to create a new Macro frame)"
        n149 = call <vilib>:"Add State(s) to Queue__JKI_lib_State_Machine.vi"("State(s) in (\"\")"=w397) -> ("States Out"=w396:string)  [unwired: 14 in]
      }
      frame "Macro: Initialize" {
        n150 = call <vilib>:"Add State(s) to Queue__JKI_lib_State_Machine.vi"("State(s) in Front (\"\")"="Data: Initialize\nInitialize Core Data\ninit Acquisition Loop\nLaunch Handshake", "State(s) in (\"\")"=w402) -> ("States Out"=w401:string)  [unwired: 13 in]
      }
      frame "Macro: Exit" {
        n151 = Unbundle By Name(w412) -> ("Core.Close Panel on Exit?"=w411:bool)
        n152 = Flush Event Queue(0:w403, 3:w405) -> (11:w404:errorcluster)  [unwired: 4 in, 2 out]
        n153 = Select(t="UI: Front Panel State >> Close", s=w411, f="") -> (s? t:f=w406:string)
        n154 = call <vilib>:"Add State(s) to Queue__JKI_lib_State_Machine.vi"("State(s) in (\"\")"=w406, "State(s) at Back (\"\")"="Exit Acquisition Loop \nData: Cleanup\nExit") -> ("States Out"=w407:string)  [unwired: 13 in]
        n155 = call <vilib>:"Add State(s) to Queue__JKI_lib_State_Machine.vi"("State(s) in Front (\"\")"=w407, "State(s) in (\"\")"=w414) -> ("States Out"=w413:string)  [unwired: 13 in]
      }
      frame "---------- Launch ----------" {
        n156 = call <vilib>:"Add State(s) to Queue__JKI_lib_State_Machine.vi"("State(s) in (\"\")"=w418) -> ("States Out"=w417:string)  [unwired: 14 in]
      }
      frame "Launch Handshake" {
        n157 = call <vilib>:"Read Self Enqueuer.vi"("Actor"=w421) -> ("Self Enqueuer"=w426:refnum<class "Message Enqueuer.lvclass">)  [unwired: 10 in]
        n158 = call <vilib>:"Read Caller Enqueuer.vi"("Actor"=w421) -> ("Caller Enqueuer"=w420:refnum<class "Message Enqueuer.lvclass">)  [unwired: 10 in]
        n159 = property class="VI"(error in=w424) -> (error out=w423:errorcluster, "Name"=w427:string)  [unwired: 1 in, 1 out]
        n160 = Bundle By Name(cluster=T12 {"Nested enqueuer"=refnum, "Clone name"=""} ("Child launch Check"), "Nested enqueuer"=w426, "Clone name"=w427) -> (w419:T12)
        n161 = call "Send Child Handshake CC.vi"("error in (no error)"=w423, "Child Core Data"=w419, "Message Enqueuer"=w420) -> ("error out"=w422:errorcluster)  [unwired: 7 in, 1 out]
        n162 = call <vilib>:"Add State(s) to Queue__JKI_lib_State_Machine.vi"("State(s) in (\"\")"=w430) -> ("States Out"=w429:string)  [unwired: 14 in]
      }
      frame "---------- State ----------" {
        n163 = call <vilib>:"Add State(s) to Queue__JKI_lib_State_Machine.vi"("State(s) in (\"\")"=w434) -> ("States Out"=w433:string)  [unwired: 14 in]
      }
      frame "Camera Info" {
        n164 = call <vilib>:"Read Caller Enqueuer.vi"("Actor"=w445) -> ("Caller Enqueuer"=w444:refnum<class "Message Enqueuer.lvclass">)  [unwired: 10 in]
        n165 = Unbundle By Name(w442) -> ("ReceiverSequence"=w438:cluster{"ReceiverID":i32, "Index":i32}[], "Camera parameters.Camera parameters.Type"=w441:string, "Exposure Time"=w435:u32, "AOI"=w440:i32[])
        n166 = Index Array(array=w438) -> (element=w439:cluster{"ReceiverID":i32, "Index":i32})  [unwired: 1 in]
        n167 = Unbundle By Name(w439) -> ("Index"=w437:i32)
        n168 = Bundle By Name(cluster=T13 {"Camera Id"=0, "Camera Name"="", "Exposure Time"=0, "AOI"=[]} ("Camera Information"), "Camera Id"=w437, "Camera Name"=w441, "Exposure Time"=w435, "AOI"=w440) -> (w436:T13)
        n169 = call "Send Camera Information CC.vi"("error in (no error)"=w447, "Camera Information"=w436, "Message Enqueuer"=w444) -> ("error out"=w446:errorcluster)  [unwired: 7 in, 1 out]
        n170 = call <vilib>:"Add State(s) to Queue__JKI_lib_State_Machine.vi"("State(s) in (\"\")"=w449) -> ("States Out"=w448:string)  [unwired: 14 in]
      }
      frame "Part Selected" {
        n171 = in-place {
          in-place-border: w459 -> [w478]
          in-place-border: w457 -> [w468]
          in-place-border: [w465] -> w456
          w469 = 0
          n172 = in-place-cluster #4(w454) -> ("Camera parameters.Camera parameters.PartsList"=w476:T17, "Camera parameters.PartName"=w475:string[], "IMAQ Run image Buffer"=w464:T1[], "IMAQ Offline Image Buffer"=w463:T1[], "Imaqdx Session In"=w462:T3, "Camera parameters.Camera parameters.Offline"=w461:bool)  [unwired: 7 out]
          n173 = Search 1D Array(1D array=w475, element=w478) -> (index of element=w477:i32)  [unwired: 1 in]
          n174 = case shown="False" w461 {
            tunnel: w468 -> [w485 w490]
            tunnel: w462 -> [w486 _]
            tunnel: [w488 w490] -> w467
            frame False {
              n175 = call <vilib>:"IMAQdx Unconfigure Acquisition.vi"("error in"=w485, "Session In"=w486) -> ("error out"=w489:errorcluster, "Session Out"=w487:T3)  [unwired: 8 in]
              n176 = call <vilib>:"IMAQdx Close Camera.vi"("error in"=w489, "Session In"=w487) -> ("error out"=w488:errorcluster)  [unwired: 9 in]
            }
            frame True {
            }
          }
          n177 = Index Array(array=w476, index=w477) -> (element=w474:T18)
          n178 = Unbundle By Name(w474) -> ("filePath"=w471:string, "AOI"=w472:i32[], "ReceiverSequence"=w473:cluster{"ReceiverID":dbl, "Index":dbl}[])
          n179 = for {
            tunnel: w467 -> [w484]
            tunnel: w463 -> [w482] mode=indexing
            tunnel: [w483] -> w466
            tunnel: [w482] -> _ mode=indexing
            n180 = call "IMAQ Dispose"("Image"=w482, "error in (no error)"=w484) -> ("error out"=w483:errorcluster)  [unwired: 4 in]
          }
          n181 = for {
            tunnel: w466 -> [w481]
            tunnel: w464 -> [w479] mode=indexing
            tunnel: [w480] -> w465
            tunnel: [w479] -> _ mode=indexing
            n182 = call "IMAQ Dispose"("Image"=w479, "error in (no error)"=w481) -> ("error out"=w480:errorcluster)  [unwired: 4 in]
          }
          n183 = String To Path(string=w471) -> (path=w470:path)
          n184 = in-place-cluster #4("Camera parameters.Camera parameters.PartsList"=w476, "Camera parameters.PartName"=w475, "CurrentPartParameters"=w474, "File path to read images"=w470, "AOI"=w472, "ReceiverSequence"=w473, "Buffer count"=w469, "Image_Counter_CA"=w469, "Buffer Number"=w469, "IMAQ Run image Buffer"=w464, "IMAQ Offline Image Buffer"=w463, "Imaqdx Session In"=w462, "Camera parameters.Camera parameters.Offline"=w461) -> (w458:T2)
        }
        n185 = Unbundle By Name(w454) -> ("Camera parameters.Camera parameters.Offline"=w453:bool)
        n186 = Select(t="", s=w453, f="Set Camera Properties") -> (s? t:f=w450:string)
        n187 = call <vilib>:"Add State(s) to Queue__JKI_lib_State_Machine.vi"("State(s) in Front (\"\")"=w450, "State(s) in (\"\")"="Data: Set Buffer" ("State(s) in (\"\")")) -> ("States Out"=w460:string)  [unwired: 13 in]
      }
      frame "Run" {
        n188 = Unbundle By Name(w495) -> ("IMAQ ring Buffer"=w500:T1[], "IMAQ Run image Buffer"=w501:T1[], "IMAQ Offline Image Buffer"=w502:T1[], "Camera parameters.Camera parameters.Offline"=w503:bool, "Imaqdx Session In"=w504:T3, "File path @ Run"=w493:path)  [unwired: 1 out]
        n189 = Empty String/Path?(string/path=w493) -> (empty?=w492:bool)
        n190 = case shown="True" w492 {
          tunnel: w504 -> [w512 w532]
          tunnel: w503 -> [_ w531]
          tunnel: [w512 w530] -> w499
          tunnel: w506 -> [w511 w529]
          tunnel: [w515 w528] -> w505
          tunnel: w493 -> [w514 w527]
          tunnel: w502 -> [w513 w526]
          tunnel: w501 -> [w508 w525]
          tunnel: w500 -> [_ w524]
          tunnel: [w509 w523] -> w498
          tunnel: [w509 w522] -> w497
          tunnel: [w513 w521] -> w496
          frame False {
            n191 = for {
              N: 1 -> [_]
              tunnel: w514 -> [w519]
              tunnel: [w518] -> w509 mode=indexing
              shift-right: [w520] -> w515
              shift-left: w511 -> [w517]
              tunnel: w508 -> [w516] mode=indexing
              n192 = call "IMAQ ReadFile"("File Path"=w519, "error in (no error)"=w517, "Image"=w516) -> ("error out"=w520:errorcluster, "Image Out"=w518:T1)  [unwired: 4 in, 3 out]
            }
          }
          frame True {
            n193 = case shown="False" w531 {
              tunnel: w529 -> [w538 w541]
              tunnel: [w537 w541] -> w528
              tunnel: w532 -> [w536 w542]
              tunnel: [w535 w542] -> w530
              tunnel: w527 -> [_ _]
              tunnel: w526 -> [w533 w540]
              tunnel: w525 -> [w534 w539]
              tunnel: [w533 w540] -> w523
              tunnel: w524 -> [_ _]
              tunnel: [w534 w539] -> w522
              tunnel: [w533 w540] -> w521
              frame False {
                # "Acquisition is started for the specified session ID"
                n194 = call <vilib>:"IMAQdx Start Acquisition.vi"("error in"=w538, "Session In"=w536) -> ("error out"=w537:errorcluster, "Session Out"=w535:T3)  [unwired: 8 in]
              }
              frame True {
                # "Offline Images are already loaded into the memory"
              }
            }
          }
        }
        n195 = call <vilib>:"Add State(s) to Queue__JKI_lib_State_Machine.vi"("State(s) in (\"\")"="init Acquisition Loop\nAcquire" ("State(s) in (\"\")")) -> ("States Out"=w507:string)  [unwired: 14 in]
        n196 = Bundle By Name(cluster=w495, "Imaqdx Session In"=w499, "IMAQ ring Buffer"=w498, "IMAQ Run image Buffer"=w497, "IMAQ Offline Image Buffer"=w496) -> (w494:T2)
      }
      frame "Pause" {
        # "For Get image Loop"
        n197 = Unbundle By Name(w547) -> ("Stop Acquisition User Event"=w553:refnum<user-event>)
        n198 = Unbundle By Name(w544) -> ("Imaqdx Session In"=w549:T3, "Camera parameters.Camera parameters.Offline"=w548:bool)
        n199 = Generate User Event "Generate Stop Acqusition User Event"(priority (normal)=usereventprio."high priority", user event=w553, event data cluster=TRUE ("event data"), error in=w546) -> (error out=w550:errorcluster)  [unwired: 1 out]
        n200 = case shown="False" w548 {
          tunnel: w550 -> [w557 w558]
          tunnel: [w556 w558] -> w545
          tunnel: w549 -> [w555 _]
          frame False {
            n201 = call <vilib>:"IMAQdx Stop Acquisition.vi"("error in"=w557, "Session In"=w555) -> ("error out"=w556:errorcluster)  [unwired: 8 in, 1 out]
          }
          frame True {
          }
        }
        n202 = call <vilib>:"Add State(s) to Queue__JKI_lib_State_Machine.vi"("State(s) in (\"\")"="") -> ("States Out"=w554:string)  [unwired: 14 in]
      }
      frame "Stop" {
        n203 = Unbundle By Name(w564) -> ("Stop Acquisition User Event"=w561:refnum<user-event>)
        n204 = case shown="\"Stop\", Default" w560 {
          tunnel: [FALSE TRUE] -> w559
          frame "Stop with Exit" {
          }
          frame "Stop", Default {
          }
        }
        n205 = Unbundle By Name(w567) -> ("Camera parameters.Camera parameters.Default file path"=w568:path, "Camera parameters.Camera parameters.AOI"=w566:i32[], "Camera parameters.Camera parameters.Continuous?"=w572:T5, "Camera parameters.Camera parameters.NumberOfBuffers"=w578:i32, "Camera parameters.Camera parameters.Id"=w573:i32, "IMAQ ring Buffer"=w576:T1[], "filenames"=w577:string[], "Imaqdx Session In"=w570:T3, "Camera parameters.Camera parameters.Offline"=w571:bool)
        n206 = call <vilib>:"Read Caller Enqueuer.vi"("Actor"=w564) -> ("Caller Enqueuer"=w579:refnum<class "Message Enqueuer.lvclass">)  [unwired: 10 in]
        n207 = Generate User Event(user event=w561, event data cluster=w559, error in=w563) -> (error out=w562:errorcluster)  [unwired: 1 in, 1 out]
        n208 = case shown="True" w571 {
          tunnel: w562 -> [w599 w612]
          tunnel: w570 -> [w597 _]
          tunnel: [w602 w611] -> w581
          tunnel: w572 -> [w601 _]
          tunnel: w578 -> [w594 _]
          tunnel: [w591 w610] -> w569
          tunnel: [w595 w609] -> w574
          tunnel: w577 -> [w591 _]
          tunnel: w576 -> [w595 w608]
          tunnel: w568 -> [_ w606]
          tunnel: [w594 w603] -> w575
          tunnel: w566 -> [w588 _]
          tunnel: w573 -> [w587 _]
          tunnel: w579 -> [w586 _]
          frame False {
            n209 = call <vilib>:"IMAQdx Stop Acquisition.vi"("error in"=w599, "Session In"=w597) -> ("error out"=w598:errorcluster, "Session Out"=w596:T3)  [unwired: 8 in]
            n210 = call <vilib>:"IMAQdx Unconfigure Acquisition.vi"("error in"=w598, "Session In"=w596) -> ("error out"=w593:errorcluster, "Session Out"=w590:T3)  [unwired: 8 in]
            n211 = call "AOI config.vi"("Camera parameters.Id"=w587, "error in (no error)"=w593, "Caller Enqueuer"=w586, "AOI"=w588, "IMAQdx in"=w590) -> ("error out"=w592:errorcluster, "IMAQdx out"=w589:T3)  [unwired: 5 in]
            n212 = To Unsigned Long Integer(number=w594) -> (unsigned 32bit integer=w600:u32)
            n213 = call <vilib>:"IMAQdx Configure Acquisition.vi"("error in"=w592, "Number of Buffers"=w600, "Continuous?"=w601, "Session In"=w589) -> ("error out"=w602:errorcluster)  [unwired: 6 in, 1 out]
          }
          frame True {
            n214 = call <vilib>:"Application Directory.vi"() -> ("Application Directory"=w607:path)
            n215 = Path To String(path=w606) -> (string=w605:string)
            n216 = Build Path(base path=w607, name or relative path=w605) -> (appended path=w604:path)
            n217 = List Folder(path=w604, error in=w612) -> (filenames=w613:string[], error out=w615:errorcluster)  [unwired: 2 in, 2 out]
            n218 = Sort 1D Array ("Sort Array")(array=w613) -> (sorted array=w614:string[])
            n219 = for {
              tunnel: w604 -> [w623]
              tunnel: w614 -> [w619] mode=indexing
              shift-right: [w622] -> w611
              shift-left: w615 -> [w618]
              tunnel: [w620] -> w609 mode=indexing
              tunnel: [w619] -> w610 mode=indexing
              tunnel: w608 -> [w617] mode=indexing
              tunnel: [w616] -> w603
              i -> [w616]
              n220 = Build Path(base path=w623, name or relative path=w619) -> (appended path=w621:path)
              n221 = call "IMAQ ReadFile"("File Path"=w621, "error in (no error)"=w618, "Image"=w617) -> ("error out"=w622:errorcluster, "Image Out"=w620:T1)  [unwired: 4 in, 3 out]
            }
          }
        }
        n222 = call <vilib>:"Add State(s) to Queue__JKI_lib_State_Machine.vi"("State(s) in (\"\")"=w583) -> ("States Out"=w582:string)  [unwired: 14 in]
        n223 = Bundle By Name(cluster=w567, "Camera parameters.Camera parameters.Timeout"=-1, "File path to read images"=w568, "AOI"=w566, "Number Of Buffers"=w575, "IMAQ ring Buffer"=w574, "filenames"=w569) -> (w580:T2)
      }
      frame "---------- Camera Settings ----------" {
        n224 = call <vilib>:"Add State(s) to Queue__JKI_lib_State_Machine.vi"("State(s) in (\"\")"=w627) -> ("States Out"=w626:string)  [unwired: 14 in]
      }
      frame "Set Camera Properties" {
        n225 = Unbundle By Name(w630) -> ("Camera parameters.Camera parameters.Continuous?"=w632:T5, "Camera parameters.Camera parameters.NumberOfBuffers"=w633:i32, "AOI"=w637:i32[], "Camera parameters"=w638:T4, "Imaqdx Session In"=w643:T3)
        n226 = call <vilib>:"Read Caller Enqueuer.vi"("Actor"=w640) -> ("Caller Enqueuer"=w639:refnum<class "Message Enqueuer.lvclass">)  [unwired: 10 in]
        n227 = call <vilib>:"IMAQdx Open Camera.vi"("error in"=w644, "Session In"=w643) -> ("error out"=w642:errorcluster, "Session Out"=w641:T3)  [unwired: 8 in]
        n228 = call "CameraConfig.vi"("AOI"=w637, "error in"=w642, "Caller Enqueuer"=w639, "ImageAcquisitionsParameters"=w638, "Session In"=w641) -> ("error out"=w635:errorcluster, "IMAQdx Session Out"=w636:T3)  [unwired: 5 in]
        n229 = To Unsigned Long Integer(number=w633) -> (unsigned 32bit integer=w631:u32)
        n230 = call <vilib>:"IMAQdx Configure Acquisition.vi"("error in"=w635, "Number of Buffers"=w631, "Continuous?"=w632, "Session In"=w636) -> ("error out"=w634:errorcluster, "Session Out"=w628:T3)  [unwired: 6 in]
        n231 = Bundle By Name(cluster=w630, "Imaqdx Session In"=w628) -> (w629:T2)
        n232 = call <vilib>:"Add State(s) to Queue__JKI_lib_State_Machine.vi"("State(s) in (\"\")"=w646) -> ("States Out"=w645:string)  [unwired: 14 in]
      }
      frame "Overwrite Camera Settings" {
        w661 = cluster{"State":string, "Status":string} {"State"="Setup", "Status"="Done"}  # State Ack
        n233 = Unbundle By Name(w663) -> ("Camera parameters.Camera parameters.Continuous?"=w666:T5, "Camera parameters.Camera parameters.NumberOfBuffers"=w667:i32, "Camera parameters.Camera parameters.GeneralCameraConfig"=w654:T15, "Imaqdx Session In"=w671:T3, "Exposure Time"=w648:u32)
        n234 = call <vilib>:"IMAQdx Stop Acquisition.vi"("error in"=w672, "Session In"=w671) -> ("error out"=w677:errorcluster, "Session Out"=w676:T3)  [unwired: 8 in]
        n235 = Index Array(array=w654, index=1) -> (element=w669:T16)
        n236 = Index Array(array=w654, index=2) -> (element=w656:T16)
        n237 = Unbundle By Name(w669) -> ("Value"=w668:string)
        n238 = call <vilib>:"IMAQdx Unconfigure Acquisition.vi"("error in"=w677, "Session In"=w676) -> ("error out"=w674:errorcluster, "Session Out"=w675:T3)  [unwired: 8 in]
        n239 = Unbundle By Name(w656) -> ("Value"=w655:string)
        n240 = case shown="\"Off\"" w668 {
          tunnel: w675 -> [w682 w685]
          tunnel: w674 -> [w681 w688]
          tunnel: [w682 w687] -> w673
          tunnel: [w681 w686] -> w662
          tunnel: w648 -> [_ w683]
          frame "On", Default {
          }
          frame "Off" {
            n241 = property class="IMAQdx"(reference=w685, error in=w688, "ActiveAttribute"="Exposure Time", "ValueU32"=w683) -> (reference out=w687:T3, error out=w686:errorcluster)
          }
        }
        n242 = Decimal String To Number(string=w655) -> (offset past number=w647:i32)  [unwired: 2 in, 1 out]
        n243 = To Unsigned Long Integer(number=w667) -> (unsigned 32bit integer=w678:u32)
        n244 = call <vilib>:"IMAQdx Configure Acquisition.vi"("error in"=w662, "Number of Buffers"=w678, "Continuous?"=w666, "Session In"=w673) -> ("error out"=w650:errorcluster, "Session Out"=w665:T3)  [unwired: 6 in]
        n245 = Select(t=w648, s=w650, f=w647) -> (s? t:f=w649:u32)
        n246 = Select(t=w661, s=w650, f=cluster{"State":string, "Status":string} {"State"="Setup", "Status"="Fail"} ("State Ack")) -> (s? t:f=w651:cluster{"State":string, "Status":string})
        n247 = Select(t="Status Update" ("f"), s=w650, f="Overwrite Camera Settings") -> (s? t:f=w659:string)
        n248 = Bundle By Name(cluster=w663, "Exposure Time"=w649, "Imaqdx Session In"=w665, "State Ack"=w651) -> (w664:T2)
        n249 = call <vilib>:"Add State(s) to Queue__JKI_lib_State_Machine.vi"("State(s) in Front (\"\")"=w659, "State(s) in (\"\")"=w680) -> ("States Out"=w679:string)  [unwired: 13 in]
      }
      frame "----------To Acquisition Loop ----------" {
        n250 = call <vilib>:"Add State(s) to Queue__JKI_lib_State_Machine.vi"("State(s) in (\"\")"=w692) -> ("States Out"=w691:string)  [unwired: 14 in]
      }
      frame "Status Update" {
        n251 = call <vilib>:"Read Caller Enqueuer.vi"("Actor"=w696) -> ("Caller Enqueuer"=w695:refnum<class "Message Enqueuer.lvclass">)  [unwired: 10 in]
        n252 = Unbundle By Name(w694) -> ("State Ack"=w693:cluster{"State":string, "Status":string})
        n253 = call "Send State Acknowledgment CC.vi"("error in (no error)"=errorcluster {"status"=FALSE, "code"=0, "source"=""}, "State Ack"=w693, "Message Enqueuer"=w695) -> ("error out"=w697:errorcluster)  [unwired: 7 in, 1 out]
        n254 = call <vilib>:"Add State(s) to Queue__JKI_lib_State_Machine.vi"("State(s) in (\"\")"=w700) -> ("States Out"=w699:string)  [unwired: 14 in]
      }
      frame "init Acquisition Loop" {
        n255 = Unbundle By Name(w707) -> ("Initialize Acquisition User Event"=w704:refnum<user-event>)
        n256 = Bundle By Name(cluster=cluster{"Initialization Data IA":T2} {"Initialization Data IA"={"Core"={"Current VI Reference"=refnum, "Close Panel on Exit?"=FALSE}, "IA JSON File Path"=path "", "Buffer Number"=0, "Missed Frame Count"=0, "Timeout"=0, "Image_Counter_CA"=0, "Imaqdx Session In"="", "filenames"=[], "File path to read images"=path "", "Sequence"="", "IMAQ ring Buffer"=[], "Buffer count"=0, "AOI"=[], "Offline Images Ring Buffer"=[], "ReceiverSequence"=[], "Number Of Buffers"=0, "IMAQ Offline Image Buffer"=[], "IMAQ Run image Buffer "=[], "Camera parameters"={"Camera parameters"={"Id"=0, "Type"="", "Model"="", "InterfaceType"="", "SerialNumber"="", "Timeout"=0, "NumberOfBuffers"=0, "AcquisitionTimeout"=0, "ImageName"="", "ColorCameraParam"={"PixelFormat"="", "GammaEnable"=FALSE, "GammaSelector"="", "BalanceRationSelector"=[], "BalanceRationRaw"=[], "BalanceWhiteAuto"="", "LightSourceSelector"=""}, "sessionID"="", "Continuous?"=enum."One Shot", "Image Type"=0, "Buffer Number Mode (Next)"=enum."Next", "PartsList"=[], "AOI "=[], "Default file path"=path "", "Offline"=FALSE, "GeneralCameraConfig"=[], "DefaultReceiverSequence"=[], "Front Panel Open?"=FALSE}, "PartName"=[]}, "CurrentPartParameters"={"Name"="", "ReceiverSequence"=[], "AOI"=[], "filePath"=""}, "Exposure Time"=0, "File path @ Run"=path "", "State Ack"={"State"="", "Status"=""}}} ("event data"), "Initialization Data IA"=w702) -> (w701:cluster{"Initialization Data IA":T2})
        n257 = Generate User Event(user event=w704, event data cluster=w701, error in=w706) -> (error out=w705:errorcluster)  [unwired: 1 in, 1 out]
        n258 = call <vilib>:"Add State(s) to Queue__JKI_lib_State_Machine.vi"("State(s) in (\"\")"=w709) -> ("States Out"=w708:string)  [unwired: 14 in]
      }
      frame "Acquire" {
        n259 = Unbundle By Name(w712) -> ("Get Image User Event"=w711:refnum<user-event>)
        n260 = Generate User Event(user event=w711, event data cluster=TRUE ("event data"), error in=w714) -> (error out=w713:errorcluster)  [unwired: 1 in, 1 out]
        n261 = call <vilib>:"Add State(s) to Queue__JKI_lib_State_Machine.vi"("State(s) in (\"\")"=w717) -> ("States Out"=w716:string)  [unwired: 14 in]
      }
      frame "Exit Acquisition loop" {
        n262 = Unbundle By Name(w721) -> ("Exit Acquisition User Event"=w720:refnum<user-event>)
        n263 = Generate User Event(priority (normal)=usereventprio."high priority", user event=w720, event data cluster=TRUE ("event data"), error in=w723) -> (error out=w722:errorcluster)  [unwired: 1 out]
        n264 = call <vilib>:"Add State(s) to Queue__JKI_lib_State_Machine.vi"("State(s) in (\"\")"=w726) -> ("States Out"=w725:string)  [unwired: 14 in]
      }
    }
  }
  n265 = call-parent "Actor Core.vi"("error in"="error in", "Actor in"="Image Acquisition in") -> ("error out"=→"error out":errorcluster, "Actor out"=→"Actor out":refnum<class "Actor.lvclass">)  [unwired: 8 in]
